vi "get voltage range ring.vi"(8 "error in (no error)":errorcluster caption="에러 입력(에러 없음)", 11 "DW7800 입력":refnum<class "DW7800.lvclass">) -> (0 "error out":errorcluster caption="에러 출력", 1 "caption":string="LDO", 2 "strings & values":T1=[{"String"="1.2V", "Value"=1.2}, {"String"="1.4V", "Value"=1.4}, {"String"="1.6V", "Value"=1.6}, {"String"="1.8V", "Value"=1.8}, {"String"="2.0V", "Value"=2.0}, {"String"="2.2V", "Value"=2.2}, {"String"="2.4V", "Value"=2.4}, {"String"="2.6V", "Value"=2.6}, {"String"="2.8V", "Value"=2.8}, {"String"="3.0V", "Value"=3.0}, {"String"="3.2V", "Value"=3.2}, {"String"="3.4V", "Value"=3.4}, {"String"="3.6V", "Value"=3.6}], 3 "DW7800 출력":refnum<class "DW7800.lvclass">, 4 "read value":dbl)   [LabVIEW 2020, in "DW7800.lvclass"]
uses:
  DW7800.lvclass
  <vilib>/Utility/miscctls.llb/LVStringsAndValuesArrayTypeDef_DBL.ctl
  Haptic IC/Haptic IC.lvclass/Haptic IC.ctl
  SubVIs/I2C/Instance VIs/(SubVI)I2C_8Bit-8Bit_Read_Single.vi
  Haptic IC/Haptic IC.lvclass
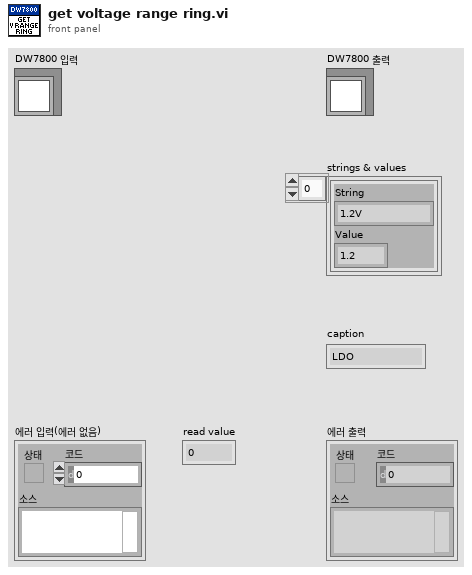
[diagram p1: front panel]
types:
  T1 = typedef "LVStringsAndValuesArrayTypeDef_DBL.ctl" = cluster{"String":string, "Value":dbl}[]
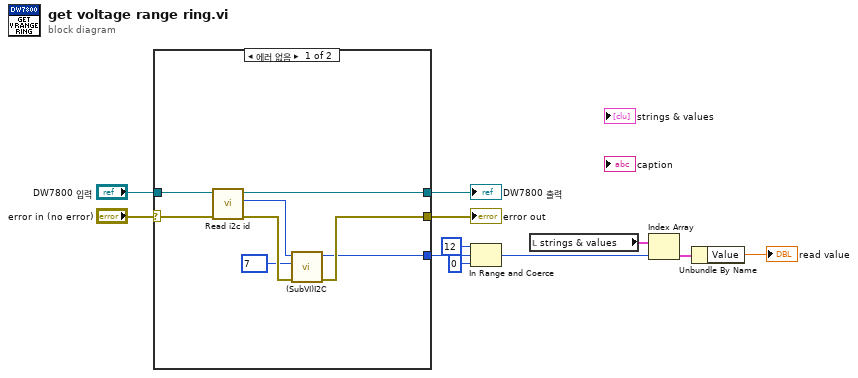
[diagram p0: block diagram]
diagram:
  n1 = case shown="에러 없음" "error in (no error)" {
    selector: "error in (no error)" -> [w18 w20]
    tunnel: "DW7800 입력" -> [w19 w21]
    tunnel: [w17 w21] -> w5
    tunnel: [w13 w20] -> w6
    tunnel: [w12 _] -> w9
    frame No Error {
      n2 = call "Read i2c id.vi"("error in (no error)"=w18, "Haptic IC 입력"=w19) -> ("error out"=w16:errorcluster, "i2c id"=w15:u8, "Haptic IC 출력"=w17:refnum<class "DW7800.lvclass">)  [unwired: 7 in]
      n3 = call-poly "(SubVI)I2C.vi"("error in (no error)"=w16, "Address"=u8 7, "ID"=w15) -> ("error out"=w13:errorcluster, "Read Data"=w12:u8)  [unwired: 6 in, 1 out]
    }
    frame Error {
    }
  }
  "error out" <- w6
  "DW7800 출력" <- w5
  n4 = In Range and Coerce(upper limit=u8 12 ("상위 리미트"), x=w9, lower limit=u8 0 ("하위 리미트")) -> (coerced(x)=w3:u8)  [unwired: 1 out]
  n5 = local read "strings & values"() -> (w10:T1)
  n6 = Index Array(array=w10, index=w3) -> (element=w11:cluster{"String":string, "Value":dbl})
  n7 = Unbundle By Name(w11) -> ("Value"=→"read value":dbl)
